vi "MessageCore.vi"(6 "Timeout (ms)":i32=-1, 8 "error in (no error)":errorcluster, 9 "Payload":string, 10 "Command":string, 11 "GRPCClient in":refnum<class "MicronGRPCClient.lvclass">) -> (0 "error out":errorcluster, 2 "Response":string, 3 "GRPCClient out":refnum<class "MicronGRPCClient.lvclass">)   [LabVIEW 2019, in "MicronGRPCClient.lvclass"]
uses:
  MicronGRPCClient.lvclass
  Generated/MicronGRPCGeneratedClient/MicronGRPCGeneratedClient.lvlib
  Generated/MicronGRPCGeneratedClient/RPC Messages/micronGrpc_MessageRequest.ctl
  06dfe680-f955-41ec-ac1b-feaf7bba287b.vi
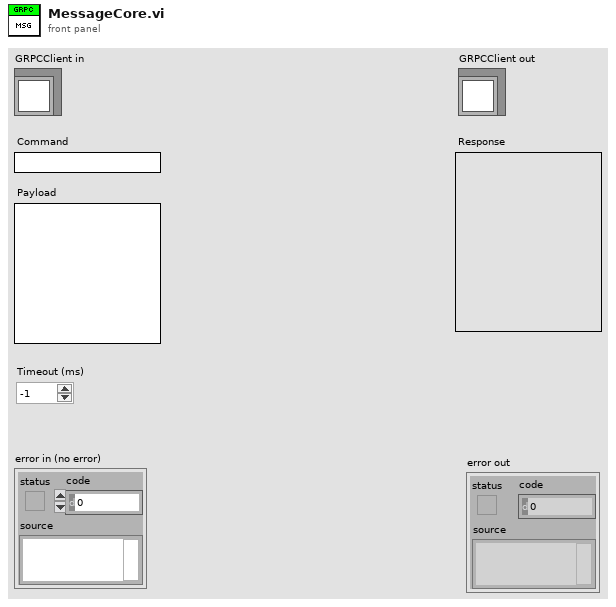
[diagram p1: front panel]
types:
  T1 = typedef "MicronGRPCGeneratedClient.lvlib/micronGrpc_MessageRequest.ctl" = cluster{"command":string, "payload":string}
  T2 = typedef "MicronGRPCClient.lvclass/gRPCDetails.ctl" = cluster{"ID":T3, "PackageName":string, "ServiceName":string, "Simulate?":bool, "ConnectionString":string, "ServiceDetails":T4}
  T3 = typedef "grpc-lvsupport-release.lvlib/grpcId.ctl" = u64
  T4 = typedef "MicronClient.lvclass/ServiceDetails.ctl" = cluster{"Micron Path":path, "Network":string, "ServiceID":string, "Port":i32, "FullyQualifiedName":string, "UI":string, "Args":string, "Mode":string, "AutoRestartOnError?":bool}
  T5 = typedef "MicronGRPCGeneratedClient.lvlib/micronGrpc_MessageReply.ctl" = cluster{"payload":string, "status":T6}
  T6 = typedef "MicronGRPCGeneratedClient.lvlib/micronGrpc_MessageReply_Status.ctl" = cluster{"code":i32, "is_error":bool, "desc":string}
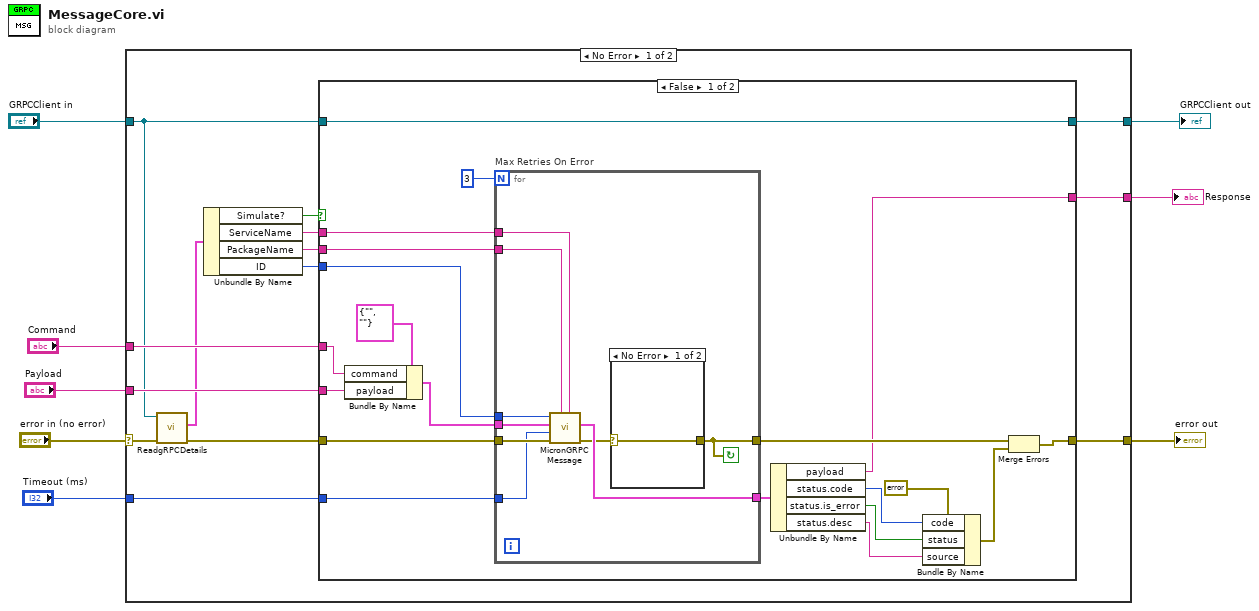
[diagram p0: block diagram]
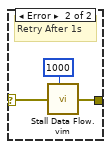
[diagram p2: hidden frame]
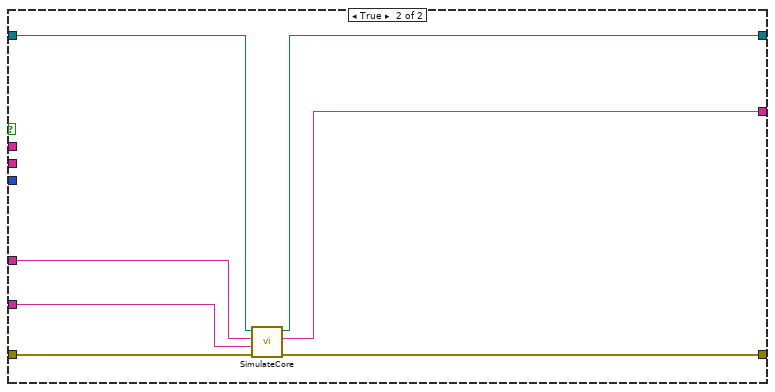
[diagram p3: hidden frame]
diagram:
  n1 = case shown="No Error" "error in (no error)" {
    selector: "error in (no error)" -> [w11 w63]
    tunnel: "GRPCClient in" -> [w10 w64]
    tunnel: "Command" -> [w17 _]
    tunnel: "Payload" -> [w16 _]
    tunnel: [w15 w63] -> w4
    tunnel: [w18 w64] -> w3
    tunnel: [w14 _] -> w2
    tunnel: "Timeout (ms)" -> [w13 _]
    frame No Error {
      n2 = call-dynamic "ReadgRPCDetails.vi"("error in (no error)"=w11, "MicronGRPCClient in"=w10) -> ("error out"=w12:errorcluster, "gRPCDetails"=w9:T2)  [unwired: 7 in, 1 out]
      n3 = Unbundle By Name(w9) -> ("Simulate?"=w19:bool, "ServiceName"=w21:string, "PackageName"=w20:string, "ID"=w22:T3)
      n4 = case shown="False" w19 {
        tunnel: w22 -> [w42 _]
        tunnel: w12 -> [w41 w62]
        tunnel: w21 -> [w39 _]
        tunnel: w20 -> [w38 _]
        tunnel: w10 -> [w37 w61]
        tunnel: [w37 w60] -> w18
        tunnel: w17 -> [w35 w59]
        tunnel: w16 -> [w34 w58]
        tunnel: [w25 w57] -> w15
        tunnel: [w24 w56] -> w14
        tunnel: w13 -> [w23 _]
        frame False {
          n5 = Bundle By Name(cluster=T1 {"command"="", "payload"=""} ("Request Data"), "command"=w35, "payload"=w34) -> (w33:T1)
          n6 = for "Max Retries On Error" {
            N: 3 -> [_]
            tunnel: w42 -> [w51]
            tunnel: [w49] -> w26
            tunnel: w33 -> [w48]
            tunnel: w41 -> [w50]
            tunnel: [w46] -> w28
            tunnel: w39 -> [w44]
            tunnel: w38 -> [w45]
            tunnel: w23 -> [w43]
            stop <- w46 continue-if-true
            n7 = call "MicronGRPC Message.vi"("Service Name"=w44, "Package Name"=w45, "error in"=w50, "timeout (ms)"=w43, "Request Data"=w48, "gRPC ID"=w51) -> ("error out"=w47:errorcluster, "Response Data"=w49:T5)  [unwired: 3 in, 1 out]
            n8 = case shown="No Error" w47 {
              selector: w47 -> [w52 w55]
              tunnel: [w52 w54] -> w46
              frame No Error {
              }
              frame Error {
                # "Retry After 1s"
                n9 = call "Stall Data Flow.vim"("value in"=w55, "milliseconds to wait"=u32 1000) -> ("value out"=w54:errorcluster)  [unwired: 1 out]
              }
            }
          }
          n10 = Unbundle By Name(w26) -> ("payload"=w24:string, "status.code"=w29:i32, "status.is_error"=w30:bool, "status.desc"=w31:string)
          n11 = Bundle By Name(cluster=errorcluster {"status"=FALSE, "code"=0, "source"=""} ("error out"), "code"=w29, "status"=w30, "source"=w31) -> (w32:errorcluster)
          n12 = Merge Errors(w28, w32) -> (w25:errorcluster)
        }
        frame True {
          n13 = call-dynamic "SimulateCore.vi"("error in (no error)"=w62, "Payload"=w58, "Command"=w59, "MicronGRPCClient in"=w61) -> ("error out"=w57:errorcluster, "Response"=w56:string, "MicronGRPCClient out"=w60:refnum<class "MicronGRPCClient.lvclass">)  [unwired: 5 in]
        }
      }
    }
    frame Error {
    }
  }
  "error out" <- w4
  "GRPCClient out" <- w3
  "Response" <- w2
